vi "Check Connection Error.vi"(8 "error in (no error)":errorcluster, 11 "TCP_Streamer_Publisher in":refnum<class "TCP_Streamer_Publisher.lvclass">) -> (0 "error out":errorcluster, 3 "TCP_Streamer_Publisher out":refnum<class "TCP_Streamer_Publisher.lvclass">)   [LabVIEW 2021, in "TCP_Streamer_Publisher.lvclass"]
uses:
  TCP_Streamer_Publisher.lvclass
  TCP_Streamer_Publisher.lvclass/TCP_Streamer_Publisher.ctl
  Typedef/State.ctl
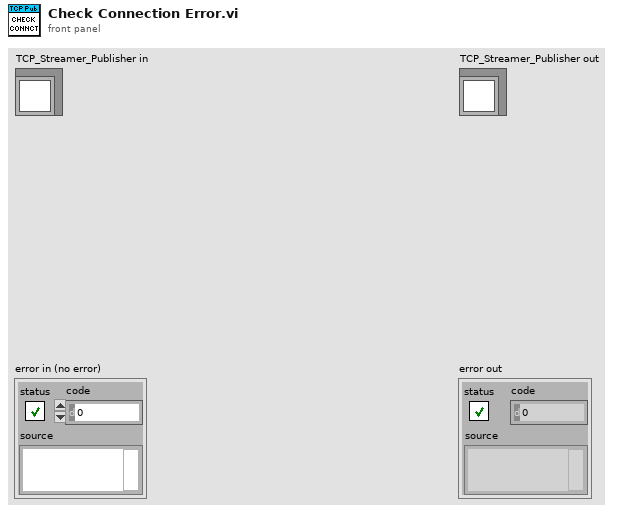
[diagram p1: front panel]
types:
  T1 = typedef "TCP_Streamer_Publisher.lvclass/State.ctl" = enum16{"Stopped", "Listening", "Ready for Data", "Ready to Send", "Sending"}
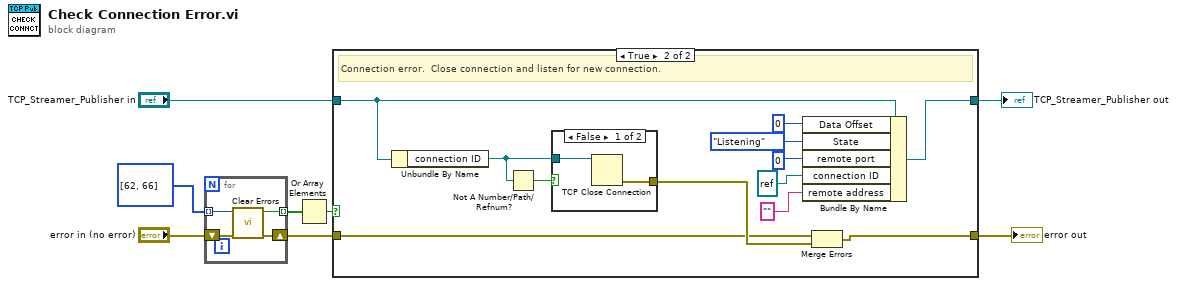
[diagram p0: block diagram]
diagram:
  n1 = for {
    tunnel: [w11] -> w2 mode=indexing
    shift-right: [w10] -> w6
    shift-left: "error in (no error)" -> [w12]
    tunnel: i32[] [62, 66] -> [w9] mode=indexing
    n2 = call <vilib>:"Clear Errors.vi"("error in (no error)"=w12, "specific error code to clear (0: all)"=w9) -> ("error out"=w10:errorcluster, "specific error cleared?"=w11:bool)  [unwired: 4 in]
  }
  n3 = Or Array Elements(Boolean array=w2) -> (logical OR=w1:bool)
  n4 = case shown="True" w1 {
    tunnel: "TCP_Streamer_Publisher in" -> [w14 w20]
    tunnel: w6 -> [w13 w17]
    tunnel: [w14 w15] -> w5
    tunnel: [w13 w16] -> w4
    frame False {
    }
    frame True {
      # "Connection error.  Close connection and listen for new connection."
      n5 = Unbundle By Name(w20) -> ("connection ID"=w18:refnum<k5>)
      n6 = Not A Number/Path/Refnum?(number/path/refnum=w18) -> (NaN/Path/Refnum?=w19:bool)
      n7 = case shown="False" w19 {
        tunnel: [w28 _] -> w22
        tunnel: w18 -> [w27 _]
        frame False {
          n8 = TCP Close Connection(connection ID=w27) -> (error out=w28:errorcluster)  [unwired: 2 in, 1 out]
        }
        frame True {
        }
      }
      n9 = Bundle By Name(cluster=w20, "Data Offset"=0, "State"=State."Listening", "remote port"=u16 0 ("port"), "connection ID"=refnum<k5> refnum, "remote address"="") -> (w15:refnum<class "TCP_Streamer_Publisher.lvclass">)
      n10 = Merge Errors(w17, w22) -> (w16:errorcluster)
    }
  }
  "error out" <- w4
  "TCP_Streamer_Publisher out" <- w5
